vi "Get All Items.vi"(0 "Display State In":T1, 9 "Container State":T2, 11 "error in (no error)":errorcluster) -> (4 "Display State Out":T1, 6 "All Names":string[](array[string]), 15 "error out":errorcluster)   [LabVIEW 2011, in "X Listbox-Solution.xctl"]
doc: "This is an additional method that was added to the X Listbox to facilitate integration of the X Control into the Wind Turbine #2 VI.\n\nAAL 9/09"
uses:
  X Listbox-Solution.xctl
  <vilib>/_xctls/Container State.ctl
  Abilities/X Listbox State.ctl
  <vilib>/_xctls/XControlSupport.lvlib
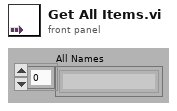
[diagram p1: front panel]
types:
  T1 = typedef "X Listbox-Solution.xctl/X Listbox State.ctl" = cluster{"# Items":i32, "Names":string[]}
  T2 = typedef "XControlSupport.lvlib/Container State.ctl" = cluster{"Indicator?":bool, "Run Mode?":bool, " Refnum":refnum<vi>}
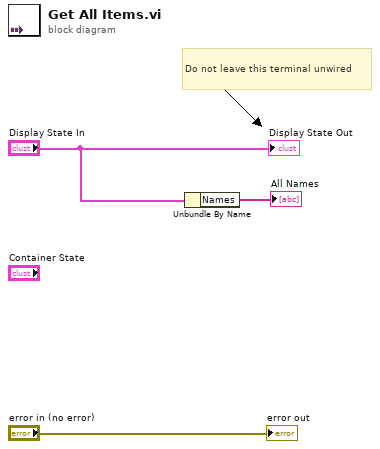
[diagram p0: block diagram]
diagram:
  # "Do not leave this terminal unwired"
  n1 = Unbundle By Name("Display State In") -> ("Names"=→"All Names":string[])
  "Display State Out" <- "Display State In"
  "error out" <- "error in (no error)"
